vi "Custom Serialization Binder.vi"() -> ()   [LabVIEW 2017]
doc: "Demonstrates the JSONtext Object Serializer by serializing a LabVIEW Object to JSON with a custom Serialization Binder."
uses:
  Generic Object Serializer/Generic Object Serializer.lvclass
  C:/Program Files (x86)/National Instruments/LabVIEW 2017/vi.lib/JDP Science/JSONtext/LVClass Serializer/JSONtext LVClass Serializer.lvclass
  Generic Object Serializer/Type Name Handling.ctl
  Account/Account.lvclass
  Generic Object Serializer/Generic Object Serializer.lvclass/Generic Object Serializer.ctl
  585c77a6-94ca-412b-a7e9-3a1ed3474501.vi
  0419a7ac-010c-49ed-bc4d-45f40a11e12e.vi
  Generic Object Serializer/Write Type Name Handling.vi
  Generic Object Serializer/Write Serialization Binder.vi
  Known Types Binder/Known Types Binder.lvclass
  C:/Users/de200256/Code/logmanoriginal/jsontext-object-serialization/Serialization Binder/Serialization Binder.lvclass
  <vilib>/JDP Science/JSONtext/Variant to JSON Text.vi
  <vilib>/JDP Science/JSONtext/JSON text to Variant.vi
panel:
  out "Summary":string
  in  "Type Name":string="Account"
  in  "CreatedDate":timestamp=timestamp(3700276200 s since 1904-01-01)
  in  "Active":bool=TRUE
  in  "Email":string="john.doe@example.com"
  in  "Roles":string[](array[string])=["User", "Admin"]
  out "error out":errorcluster
  out "<JSON>":string
  # "Overview\nDemonstrates the JSONtext Object Serializer by serializing a LabVIEW Object to JSON with a custom Serialization Binder.\n\nInstructions\nRun the VI"
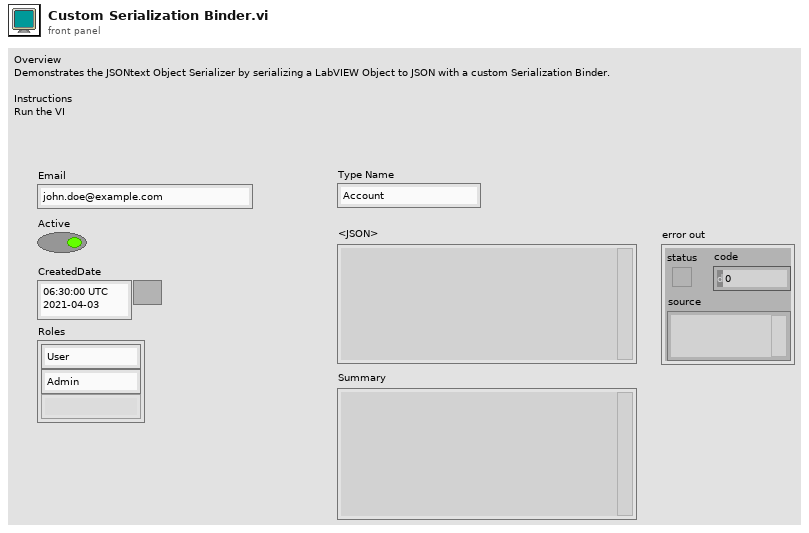
[diagram p1: front panel]
types:
  T1 = typedef "Generic Object Serializer.lvclass/Type Name Handling.ctl" = enum16{"None", "Inline"}
  T2 = typedef "Known Types Binder.lvclass/Known Type.ctl" = cluster{"Name":string, "Type":refnum<class>}
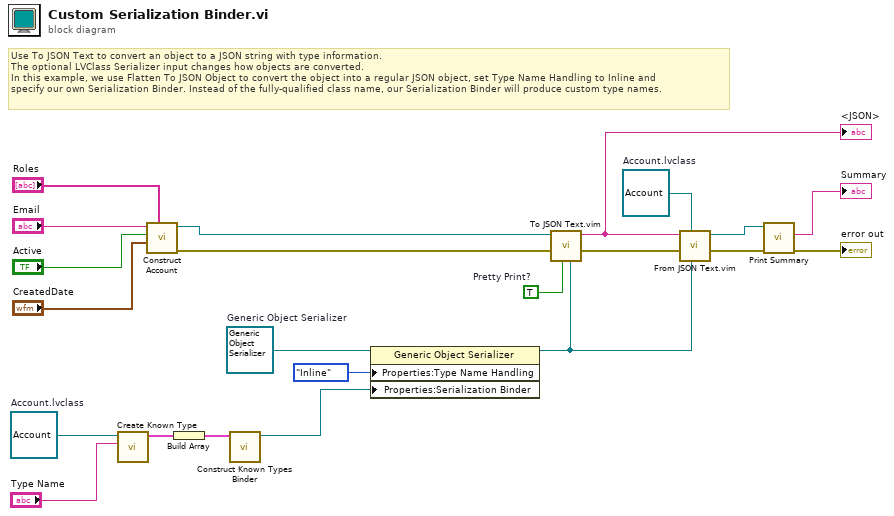
[diagram p0: block diagram]
diagram:
  w5 = refnum<class "Account.lvclass"> refnum  # Account.lvclass
  w10 = refnum<class "Account.lvclass"> refnum  # Account.lvclass
  w15 = refnum<class "Generic Object Serializer.lvclass"> refnum  # Generic Object Serializer
  w16 = TRUE  # Pretty Print?
  # "Use To JSON Text to convert an object to a JSON string with type information.\nThe optional LVClass Serializer input changes how objects are converted.\nIn this example, we use Flatten To JSON Object to convert the object into a regular JSON object, set Type Name Handling to Inline and\nspecify our own Serialization Binder. Instead of the fully-qualified class name, our Serialization Binder will produce custom type names."
  n1 = call "Create Known Type.vi"("Name"="Type Name", "Type"=w10) -> ("Known Type"=w12:T2)  [unwired: 9 in]
  n2 = call "Construct Account.vi"("Roles"="Roles", "CreatedDate"="CreatedDate", "Active"="Active", "Email"="Email") -> ("error out"=w18:errorcluster, "Account"=w17:refnum<class "Account.lvclass">)  [unwired: 6 in]
  n3 = Build Array(w12) -> (w11:T2[])
  n4 = call "Construct Known Types Binder.vi"("Known Types"=w11) -> ("Known Types Binder"=w13:refnum<class "Known Types Binder.lvclass">)  [unwired: 9 in, 1 out]
  n5 = property class="Generic Object Serializer"(reference=w15, "Properties:Type Name Handling"=Type_Name_Handling."Inline" ("Type Name Handling"), "Properties:Serialization Binder"=w13) -> (reference out=w1:refnum<class "Generic Object Serializer.lvclass">)  [unwired: 1 in, 1 out]
  n6 = call "To JSON Text.vim"("LVClass Serializer"=w1, "Pretty Print?"=w16, "error in (no error)"=w18, "Anything"=w17) -> ("error out"=w8:errorcluster, "<JSON>"=w6:string)  [unwired: 6 in]
  "<JSON>" <- w6
  n7 = call "From JSON Text.vim"("LVClass Serializer"=w1, "Data Type and Default Value"=w5, "error in (no error)"=w8, "JSON"=w6) -> ("error out"=w7:errorcluster, "Data out"=w4:refnum<class "Account.lvclass">)  [unwired: 6 in]
  n8 = call "Print Summary.vi"("error in (no error)"=w7, "Account in"=w4) -> ("error out"=→"error out":errorcluster, "Summary"=→"Summary":string)  [unwired: 7 in, 1 out]
